vi "DestroyTexture.vi"(8 "No Error":errorcluster, 11 "Texture [SDL_Texture *]":T1 format="%.0x") -> (0 "error out":errorcluster)   [LabVIEW 2026, in "SDL3.lvlib" / "Render.lvlib"]
doc: "<B>Summary</B>\nDestroy the specified texture.\n\n<B>Remarks</B>\nPassing NULL or an otherwise invalid texture will set the SDL error message to \"Invalid texture\"."
uses:
  Render.lvlib
  Lib/SDL3.dll
  SDL_Texture--pointer.ctl
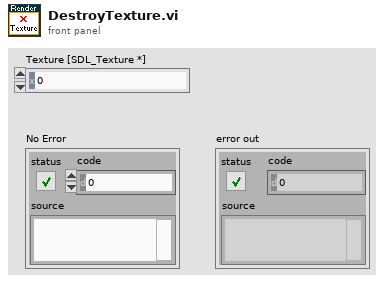
[diagram p1: front panel]
types:
  T1 = typedef "SDL3.lvlib/Render.lvlib/SDL_Texture--pointer.ctl" = i64
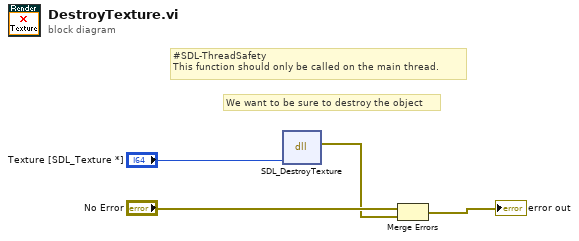
[diagram p0: block diagram]
diagram:
  # "#SDL-ThreadSafety\nThis function should only be called on the main thread."
  # "We want to be sure to destroy the object"
  n1 = dll-call lib="C:/Users/saukko/Dev/LV-SDL3/Sources/SDL3/Lib/SDL3.*" fn="SDL_DestroyTexture"("window"="Texture [SDL_Texture *]") -> (error out=w1:errorcluster)  [unwired: 5 in, 1 out]
  n2 = Merge Errors("No Error", w1) -> (→"error out":errorcluster)
